vi "calculate Chi.vi"(0 "Chi_A":dbl format="%#_13g", 1 "CO2/H2O":T1, 2 "Z":dbl, 5 "Psi_A":dbl format="%#_13g", 7 "Psi_B":dbl format="%#_13g", 9 "W_A [raw signal]":dbl format="%#_13g", 11 "W_B [raw signal]":dbl format="%#_13g", 12 "T [K]":dbl format="%#_13g", 13 "P [kPa]":dbl format="%#_13g", 14 "S":dbl=1.39327 format="%#_13g") -> (8 "Chi_B":dbl)   [LabVIEW 2017, in "LicorLI7000.lvlib"]
uses:
  LicorLI7000.lvlib
  conventions/Substance.ctl
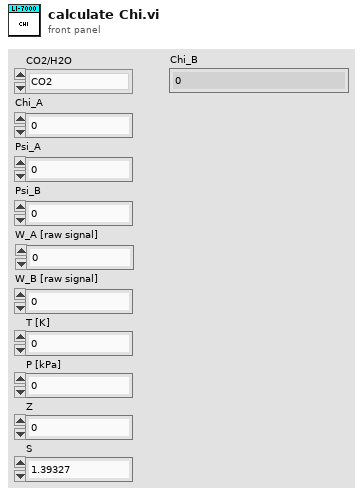
[diagram p1: front panel]
types:
  T1 = typedef "LicorLI7000.lvlib/Substance.ctl" = enum16{"CO2", "H2O"}
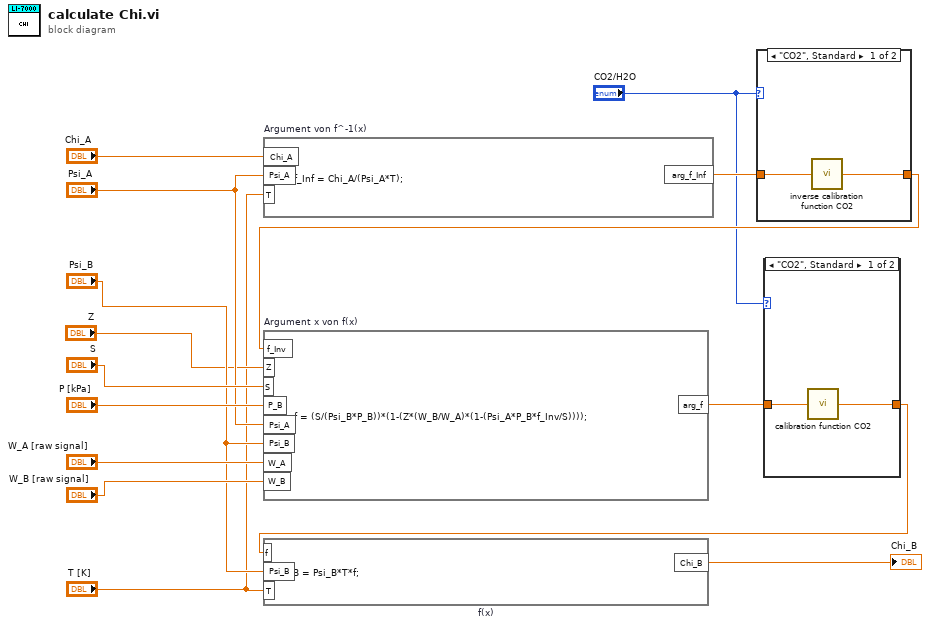
[diagram p0: block diagram]
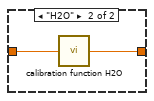
[diagram p2: hidden frame]
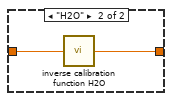
[diagram p3: hidden frame]
diagram:
  n1 = formula code="arg_f_Inf = Chi_A/(Psi_A*T);" "Argument von f^-1(x)"("Chi_A"="Chi_A", "Psi_A"="Psi_A", "T"="T [K]") -> ("arg_f_Inf"=w9:dbl)
  n2 = case shown="\"CO2\", Standard" "CO2/H2O" {
    tunnel: w9 -> [w17 w19]
    tunnel: [w16 w18] -> w8
    frame "CO2", Default {
      n3 = call "inverse calibration function CO2.vi"("x"=w17) -> ("f_inv(x)"=w16:dbl)  [unwired: 14 in]
    }
    frame "H2O" {
      n4 = call "inverse calibration function H2O.vi"("x"=w19) -> ("f_inv(x)"=w18:dbl)  [unwired: 14 in]
    }
  }
  n5 = formula code="arg_f = (S/(Psi_B*P_B))*(1-(Z*(W_B/W_A)*(1-(Psi_A*P_B*f_Inv/S))));" "Argument x von f(x)"("f_Inv"=w8, "Z"="Z", "S"="S", "P_B"="P [kPa]", "Psi_A"="Psi_A", "Psi_B"="Psi_B", "W_A"="W_A [raw signal]", "W_B"="W_B [raw signal]") -> ("arg_f"=w3:dbl)
  n6 = case shown="\"CO2\", Standard" "CO2/H2O" {
    tunnel: w3 -> [w21 w23]
    tunnel: [w20 w22] -> w2
    frame "CO2", Default {
      n7 = call "calibration function CO2.vi"("x"=w21) -> ("f(x)"=w20:dbl)  [unwired: 14 in]
    }
    frame "H2O" {
      n8 = call "calibration function H2O.vi"("x"=w23) -> ("f(x)"=w22:dbl)  [unwired: 14 in]
    }
  }
  n9 = formula code="Chi_B = Psi_B*T*f;" "f(x)"("f"=w2, "Psi_B"="Psi_B", "T"="T [K]") -> ("Chi_B"=→"Chi_B":dbl)
